vi "Variant_to_Cluster.vi"(8 "Error in":errorcluster, 11 "Value (in)":variant) -> (0 "Error out":errorcluster, 2 "Value (string)":string, 3 "Value (out)":string)   [LabVIEW 2012]
uses:
  Variant_to_I8.vi
  Variant_to_I16.vi
  Variant_to_I32.vi
  Variant_to_I64.vi
  Variant_to_U8.vi
  Variant_to_U16.vi
  Variant_to_U32.vi
  Variant_to_U64.vi
  Variant_to_SGL.vi
  Variant_to_DBL.vi
  Variant_to_EXT.vi
  Variant_to_CSG.vi
  Variant_to_CDB.vi
  Variant_to_CXT.vi
  Variant_to_Enum_U8.vi
  Variant_to_Enum_U16.vi
  Variant_to_Enum_U32.vi
  Variant_to_Enum_U64.vi
  Variant_to_Boolean.vi
  Variant_to_String.vi
  Variant_to_Path.vi
  Variant_to_Array.vi
  Variant_to_Waveform_info.vi
  Variant_to_Timestamp.vi
  Variant_to_Refnum.vi
  Variant_to_Fixed_point.vi
  <vilib>/Utility/VariantDataType/VariantType.lvlib
  Variant_to_Waveform.vi
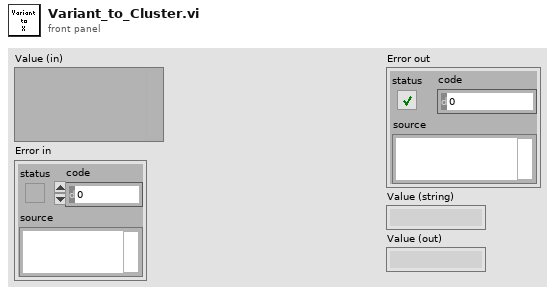
[diagram p1: front panel]
types:
  T1 = typedef "VariantType.lvlib/Type.ctl" = enum8{"Invalid Type", "Void", "I8", "I16", "I32", "I64", "U8", "U16", "U32", "U64", "Single Float", "Double Float", "Extended Float", "Single Complex", "Double Complex", "Extended Complex", "Enum U8", "Enum U16", "Enum U32", "Enum U64", "Single Float With Unit", "Double Float With Unit", "Extended Float With Unit", "Single Complex with Unit", "Double Complex with Unit", "Extended Complex with Unit", "Boolean", "String", "Path", "Picture", "Tag", "Array", "Cluster", "Variant", "LV Variant", "Waveform", "Timestamp", "Digital Waveform", "Digital Data", "ExpressData", "Refnum", "External Data", "VI", "Poly VI", "LabVIEW Class Instance", "Fixed Point"}
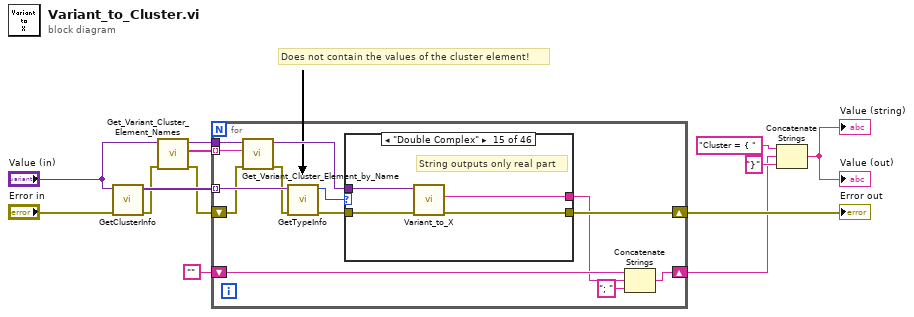
[diagram p0: block diagram]
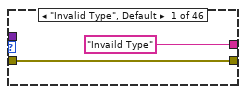
[diagram p2: hidden frame]
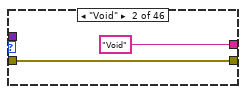
[diagram p3: hidden frame]
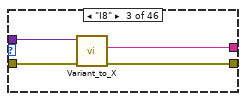
[diagram p4: hidden frame]
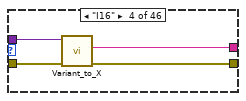
[diagram p5: hidden frame]
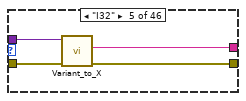
[diagram p6: hidden frame]
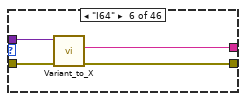
[diagram p7: hidden frame]
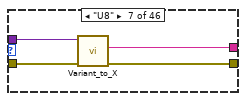
[diagram p8: hidden frame]
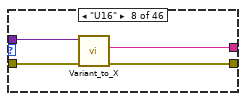
[diagram p9: hidden frame]
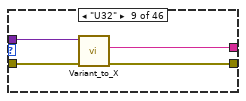
[diagram p10: hidden frame]
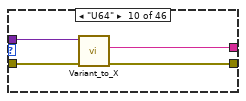
[diagram p11: hidden frame]
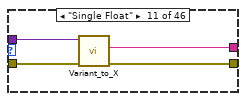
[diagram p12: hidden frame]
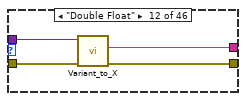
[diagram p13: hidden frame]
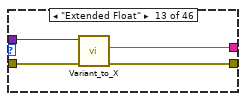
[diagram p14: hidden frame]
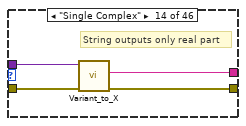
[diagram p15: hidden frame]
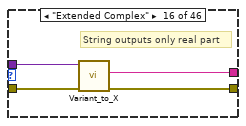
[diagram p16: hidden frame]
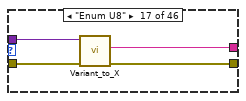
[diagram p17: hidden frame]
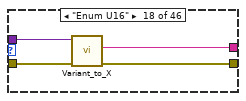
[diagram p18: hidden frame]
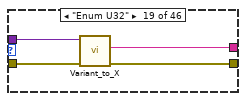
[diagram p19: hidden frame]
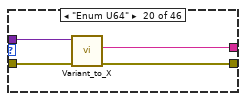
[diagram p20: hidden frame]
diagram:
  # "Does not contain the values of the cluster element!"
  n1 = call <vilib>:"GetClusterInfo.vi"("error in (no error)"="Error in", "Variant"="Value (in)") -> ("error out"=w4:errorcluster, "Cluster Elements"=w6:variant[])  [unwired: 8 in]
  n2 = call "Get_Variant_Cluster_Element_Names.vi"("error in (no error)"=w4, "Cluster in"="Value (in)") -> ("error out"=w2:errorcluster, "Element names"=w3:string[], "Cluster out"=w1:variant)  [unwired: 7 in]
  n3 = for {
    tunnel: w6 -> [w22] mode=indexing
    shift-right: [w21] -> w11
    shift-left: w2 -> [w15]
    shift-right: [w24] -> w8
    shift-left: "" -> [w26]
    tunnel: w3 -> [w18] mode=indexing
    tunnel: w1 -> [w14]
    n4 = call "Get_Variant_Cluster_Element_by_Name.vi"("error in (no error)"=w15, "Element name"=w18, "Cluster"=w14) -> ("error out"=w16:errorcluster, "VElement"=w17:variant)  [unwired: 6 in, 1 out]
    n5 = call <vilib>:"GetTypeInfo.vi"("error in (no error)"=w16, "Variant"=w22) -> ("error out"=w23:errorcluster, "Type Enum"=w19:T1)  [unwired: 5 in, 3 out]
    n6 = case shown="\"Double Complex\"" w19 {
      tunnel: ["Invaild Type" "Void" w32 w35 w39 w43 w47 w51 w55 w60 w64 w67 w71 w75 w79 w83 w87 w92 w95 w99 "{Single Float With Unit}" "{Double Float With Unit}" "{Extended Float With Unit}" "{Single Complex with Unit}" "{Double Complex with Unit}" "{Extended Complex with Unit}" w115 w119 w123 "{Picture}" "{Tag}" w131 w135 "{Variant}" "{LV Variant}" w143 w155 "{Digital Wavefrom}" "{Digital Data}" "{ExpressData}" w165 "{External Data}" "{VI}" "{Poly VI}" "{LabVIEW Class Instance}" w177] -> w20
      tunnel: w17 -> [_ _ w34 w38 w42 w46 w50 w54 w58 w62 w66 w68 w74 w78 w82 w84 w90 w94 w98 w102 _ _ _ _ _ _ w118 w122 w126 _ _ w132 w138 _ _ w146 w158 _ _ _ w168 _ _ _ _ w180]
      tunnel: w23 -> [w27 w29 w33 w37 w41 w45 w49 w53 w57 w61 w65 w70 w73 w77 w81 w86 w89 w93 w97 w101 w104 w106 w108 w110 w112 w114 w117 w121 w125 w128 w130 w134 w137 w140 w142 w145 w157 w159 w162 w164 w167 w170 w172 w174 w176 w179]
      tunnel: [w27 w29 w31 w36 w40 w44 w48 w52 w56 w59 w63 w69 w72 w76 w80 w85 w88 w91 w96 w100 w104 w106 w108 w110 w112 w114 w116 w120 w124 w128 w130 w133 w136 w140 w142 w144 w156 w159 w162 w164 w166 w170 w172 w174 w176 w178] -> w21
      frame "Invalid Type", Default {
      }
      frame "Void" {
      }
      frame "I8" {
        n7 = call-poly "Variant_to_X.vi"("Error in"=w33, "Value (in)"=w34) -> ("Error out"=w31:errorcluster, "Value (string)"=w32:string)  [unwired: 7 in, 1 out]
      }
      frame "I16" {
        n8 = call-poly "Variant_to_X.vi"("Error in"=w37, "Value (in)"=w38) -> ("Error out"=w36:errorcluster, "Value (string)"=w35:string)  [unwired: 7 in, 1 out]
      }
      frame "I32" {
        n9 = call-poly "Variant_to_X.vi"("Error in"=w41, "Value (in)"=w42) -> ("Error out"=w40:errorcluster, "Value (string)"=w39:string)  [unwired: 7 in, 1 out]
      }
      frame "I64" {
        n10 = call-poly "Variant_to_X.vi"("Error in"=w45, "Value (in)"=w46) -> ("Error out"=w44:errorcluster, "Value (string)"=w43:string)  [unwired: 7 in, 1 out]
      }
      frame "U8" {
        n11 = call-poly "Variant_to_X.vi"("Error in"=w49, "Value (in)"=w50) -> ("Error out"=w48:errorcluster, "Value (string)"=w47:string)  [unwired: 7 in, 1 out]
      }
      frame "U16" {
        n12 = call-poly "Variant_to_X.vi"("Error in"=w53, "Value (in)"=w54) -> ("Error out"=w52:errorcluster, "Value (string)"=w51:string)  [unwired: 7 in, 1 out]
      }
      frame "U32" {
        n13 = call-poly "Variant_to_X.vi"("Error in"=w57, "Value (in)"=w58) -> ("Error out"=w56:errorcluster, "Value (string)"=w55:string)  [unwired: 7 in, 1 out]
      }
      frame "U64" {
        n14 = call-poly "Variant_to_X.vi"("Error in"=w61, "Value (in)"=w62) -> ("Error out"=w59:errorcluster, "Value (string)"=w60:string)  [unwired: 7 in, 1 out]
      }
      frame "Single Float" {
        n15 = call-poly "Variant_to_X.vi"("Error in"=w65, "Value (in)"=w66) -> ("Error out"=w63:errorcluster, "Value (string)"=w64:string)  [unwired: 7 in, 1 out]
      }
      frame "Double Float" {
        n16 = call-poly "Variant_to_X.vi"("Error in"=w70, "Value (in)"=w68) -> ("Error out"=w69:errorcluster, "Value (string)"=w67:string)  [unwired: 7 in, 1 out]
      }
      frame "Extended Float" {
        n17 = call-poly "Variant_to_X.vi"("Error in"=w73, "Value (in)"=w74) -> ("Error out"=w72:errorcluster, "Value (string)"=w71:string)  [unwired: 7 in, 1 out]
      }
      frame "Single Complex" {
        # "String outputs only real part"
        n18 = call-poly "Variant_to_X.vi"("Error in"=w77, "Value (in)"=w78) -> ("Error out"=w76:errorcluster, "Value (string)"=w75:string)  [unwired: 7 in, 1 out]
      }
      frame "Double Complex" {
        # "String outputs only real part"
        n19 = call-poly "Variant_to_X.vi"("Error in"=w81, "Value (in)"=w82) -> ("Error out"=w80:errorcluster, "Value (string)"=w79:string)  [unwired: 7 in, 1 out]
      }
      frame "Extended Complex" {
        # "String outputs only real part"
        n20 = call-poly "Variant_to_X.vi"("Error in"=w86, "Value (in)"=w84) -> ("Error out"=w85:errorcluster, "Value (string)"=w83:string)  [unwired: 7 in, 1 out]
      }
      frame "Enum U8" {
        n21 = call-poly "Variant_to_X.vi"("Error in"=w89, "Value (in)"=w90) -> ("Error out"=w88:errorcluster, "Value (string)"=w87:string)  [unwired: 7 in, 1 out]
      }
      frame "Enum U16" {
        n22 = call-poly "Variant_to_X.vi"("Error in"=w93, "Value (in)"=w94) -> ("Error out"=w91:errorcluster, "Value (string)"=w92:string)  [unwired: 7 in, 1 out]
      }
      frame "Enum U32" {
        n23 = call-poly "Variant_to_X.vi"("Error in"=w97, "Value (in)"=w98) -> ("Error out"=w96:errorcluster, "Value (string)"=w95:string)  [unwired: 7 in, 1 out]
      }
      frame "Enum U64" {
        n24 = call-poly "Variant_to_X.vi"("Error in"=w101, "Value (in)"=w102) -> ("Error out"=w100:errorcluster, "Value (string)"=w99:string)  [unwired: 7 in, 1 out]
      }
      frame "Single Float With Unit" {
      }
      frame "Double Float With Unit" {
      }
      frame "Extended Float With Unit" {
      }
      frame "Single Complex with Unit" {
      }
      frame "Double Complex with Unit" {
      }
      frame "Extended Complex with Unit" {
      }
      frame "Boolean" {
        n25 = call-poly "Variant_to_X.vi"("Error in"=w117, "Value (in)"=w118) -> ("Error out"=w116:errorcluster, "Value (string)"=w115:string)  [unwired: 7 in, 1 out]
      }
      frame "String" {
        n26 = call-poly "Variant_to_X.vi"("Error in"=w121, "Value (in)"=w122) -> ("Error out"=w120:errorcluster, "Value (string)"=w119:string)  [unwired: 7 in, 1 out]
      }
      frame "Path" {
        n27 = call-poly "Variant_to_X.vi"("Error in"=w125, "Value (in)"=w126) -> ("Error out"=w124:errorcluster, "Value (string)"=w123:string)  [unwired: 7 in, 1 out]
      }
      frame "Picture" {
      }
      frame "Tag" {
      }
      frame "Array" {
        n28 = call-poly "Variant_to_X.vi"("Error in"=w134, "Value (in)"=w132) -> ("Error out"=w133:errorcluster, "Value (string)"=w131:string)  [unwired: 7 in, 1 out]
      }
      frame "Cluster" {
        n29 = call-poly "Variant_to_X.vi"("Error in"=w137, "Value (in)"=w138) -> ("Error out"=w136:errorcluster, "Value (string)"=w135:string)  [unwired: 7 in, 1 out]
      }
      frame "Variant" {
      }
      frame "LV Variant" {
      }
      frame "Waveform" {
        n30 = disable-structure shown="Enabled" {
          disable-tunnel: w146 -> [w150 w154]
          disable-tunnel: w145 -> [w149 w153]
          disable-tunnel: [w148 w152] -> w144
          disable-tunnel: [w147 w151] -> w143
          frame Disabled {
            n31 = call-poly "Variant_to_X.vi"("Error in"=w149, "Value (in)"=w150) -> ("Error out"=w148:errorcluster, "Value (string)"=w147:string)  [unwired: 7 in, 1 out]
          }
          frame Enabled {
            n32 = call-poly "Variant_to_X.vi"("Error in"=w153, "Value (in)"=w154) -> ("Error out"=w152:errorcluster, "Value (string)"=w151:string)  [unwired: 7 in, 1 out]
          }
        }
      }
      frame "Timestamp" {
        n33 = call-poly "Variant_to_X.vi"("Error in"=w157, "Value (in)"=w158) -> ("Error out"=w156:errorcluster, "Value (string)"=w155:string)  [unwired: 7 in, 1 out]
      }
      frame "Digital Waveform" {
      }
      frame "Digital Data" {
      }
      frame "ExpressData" {
      }
      frame "Refnum" {
        n34 = call-poly "Variant_to_X.vi"("Error in"=w167, "Value (in)"=w168) -> ("Error out"=w166:errorcluster, "Value (string)"=w165:string)  [unwired: 5 in, 3 out]
      }
      frame "External Data" {
      }
      frame "VI" {
      }
      frame "Poly VI" {
      }
      frame "LabVIEW Class Instance" {
      }
      frame "Fixed Point" {
        n35 = call-poly "Variant_to_X.vi"("Error in"=w179, "Value (in)"=w180) -> ("Error out"=w178:errorcluster, "Value (string)"=w177:string)  [unwired: 7 in, 1 out]
      }
    }
    n36 = Concatenate Strings(w26, w20, "; " ("string")) -> (w24:string)
  }
  "Error out" <- w11
  n37 = Concatenate Strings("Cluster = { " ("string"), w8, "}" ("string")) -> (→"Value (out)" →"Value (string)":string)
